vi "Format Version Number.vi"(8 "Number of Digits (4)":i32=4, 9 "Version In":string) -> (1 "Version Out":string)   [LabVIEW 2016, in "SLL Application.lvlib"]
doc: "Formats the version number to be in the required number of digits. \n\nEg: If version input is 1.0 and the number of digits is 4, then version out will be 1.0.0.0\n\nIf the number of digits is specified as -1 or 0, it will ignore the operation."
uses:
  SLL Application.lvlib
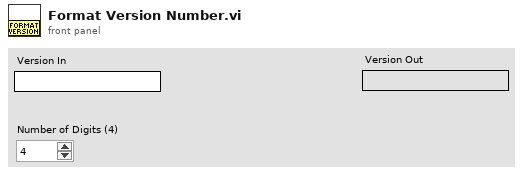
[diagram p1: front panel]
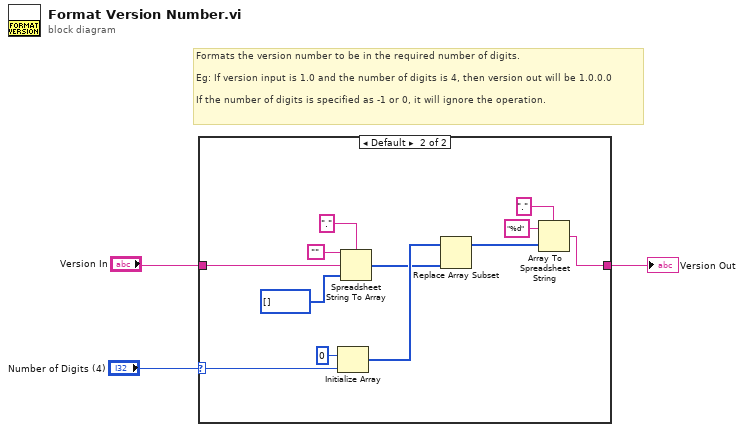
[diagram p0: block diagram]
diagram:
  # "Formats the version number to be in the required number of digits. \n\nEg: If version input is 1.0 and the number of digits is 4, then version out will be 1.0.0.0\n\nIf the number of digits is specified as -1 or 0, it will ignore the operation."
  n1 = case shown="Default" "Number of Digits (4)" {
    selector: "Number of Digits (4)" -> [_ w14]
    tunnel: [w4 w16] -> w3
    tunnel: "Version In" -> [w4 w15]
    frame -1, 0 {
      # "Retain the input version number"
    }
    frame Default {
      n2 = Initialize Array(u32 0 ("element"), w14) -> (w9:u32[])
      n3 = Spreadsheet String To Array(delimiter (Tab)=".", format string="", spreadsheet string=w15, array type (2D Dbl)=u32[] []) -> (array=w8:u32[])
      n4 = Replace Array Subset(array=w9, new element=w8) -> (w7:u32[])  [unwired: 1 in]
      n5 = Array To Spreadsheet String(delimiter (Tab)=".", array=w7, 3:"%d" ("format string")) -> (spreadsheet string=w16:string)
    }
  }
  "Version Out" <- w3
